vi "Target Address.vi"(6 "Addr. Mode":refnum<data-value>, 8 "error in (no error)":errorcluster, 11 "Low Speed in":refnum<class "Low Speed.lvclass">) -> (0 "error out":errorcluster, 3 "Low Speed out":refnum<class "Low Speed.lvclass">)   [LabVIEW 2020, in "Low Speed.lvclass"]
uses:
  Low Speed.lvclass
  C:/Users/kaiser.asan/OneDrive - SolitonTechnologies/LabVIEW/29.SDLC - I2C Driver/I2C Module/I2C Controller Module/Class/Transmission Mode/Parent/TX Speed.lvclass
  Addressing Mode/Parent/Addressing Mode.lvclass
  Parent/TX Speed.lvclass
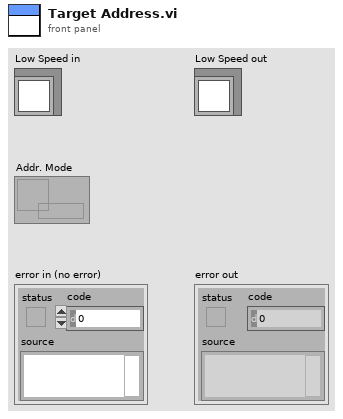
[diagram p1: front panel]
types:
  T1 = typedef "I2C Controller Lib.lvlib/Timing Parameters Cluster.ctl" = cluster{"f_SCL(KHz)":u32, "t_HIGH (ns)":u32, "t_LOW (ns)":u32, "t_SU;STA (ns)":u32, "t_HD;STA (ns)":u32, "t_SU;DAT (ns)":u32, "t_HD;DAT (ns)":u32, "t_SU;STO (ns)":u32, "t_BUF (ns)":u32}
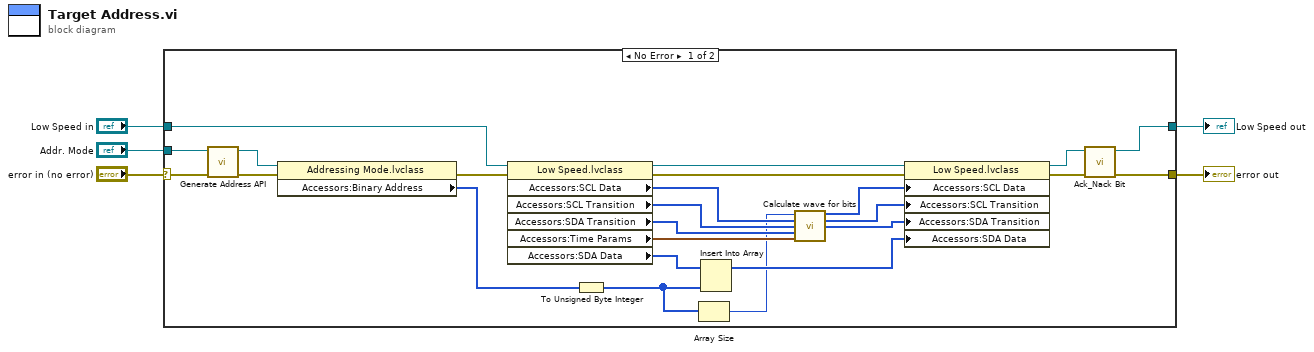
[diagram p0: block diagram]
diagram:
  n1 = case shown="No Error" "error in (no error)" {
    selector: "error in (no error)" -> [w28 w31]
    tunnel: [w8 w31] -> w5
    tunnel: [w9 w30] -> w4
    tunnel: "Low Speed in" -> [w24 w30]
    tunnel: "Addr. Mode" -> [w29 _]
    frame No Error {
      n2 = call "Generate Address API.vi"("error in (no error)"=w28, "DVR IN"=w29) -> ("error out"=w27:errorcluster, "DVR OUT"=w25:refnum<data-value>)  [unwired: 8 in]
      n3 = property class="Addressing Mode.lvclass"(reference=w25, error in=w27) -> (error out=w26:errorcluster, "Accessors:Binary Address"=w23:i16[])  [unwired: 1 out]
      n4 = property class="Low Speed.lvclass"(reference=w24, error in=w26) -> (reference out=w20:refnum<class "Low Speed.lvclass">, error out=w19:errorcluster, "Accessors:SCL Data"=w18:u8[], "Accessors:SCL Transition"=w17:u32[], "Accessors:SDA Transition"=w16:u32[], "Accessors:Time Params"=w15:T1, "Accessors:SDA Data"=w22:u8[])
      n5 = To Unsigned Byte Integer(number=w23) -> (unsigned 8bit integer=w7:u8[])
      n6 = Array Size(array=w7) -> (size(s)=w6:i32)
      n7 = Insert Into Array(array=w22, new element=w7) -> (w21:u8[])  [unwired: 1 in]
      n8 = call "Calculate wave for bits.vi"("No. Of Bits"=w6, "SCL DATA IN"=w18, "SCL Transitions In"=w17, "SDA Transitions In"=w16, "Time Params"=w15) -> ("SCL DATA OUT"=w14:u8[], "SCL Transitions Out"=w13:u32[], "SDA Transitions Out"=w12:u32[])  [unwired: 8 in]
      n9 = property class="Low Speed.lvclass"(reference=w20, error in=w19, "Accessors:SCL Data"=w14, "Accessors:SCL Transition"=w13, "Accessors:SDA Transition"=w12, "Accessors:SDA Data"=w21) -> (reference out=w10:refnum<class "Low Speed.lvclass">, error out=w11:errorcluster)
      n10 = call-dynamic "Ack_Nack Bit.vi"("error in (no error)"=w11, "Low Speed in"=w10) -> ("error out"=w8:errorcluster, "Low Speed out"=w9:refnum<class "Low Speed.lvclass">)  [unwired: 8 in]
    }
    frame Error {
    }
  }
  "error out" <- w5
  "Low Speed out" <- w4
